vi "Write Pumps Voltages.vi"(8 "error in (no error)":errorcluster, 10 "Pumps Voltages":dbl[](array[numeric]), 11 "FPGA VI Reference In":T1) -> (0 "error out":errorcluster, 3 "FPGA VI Reference Out":T1)   [LabVIEW 2018, in "RT-FPGA Interface API.lvlib"]
uses:
  RT-FPGA Interface API.lvlib
  FPGA ref.ctl
  <vilib>/Utility/error.llb/Error Cluster From Error Code.vi
  <vilib>/rvi/errors/niLvFpgaAdjustHostInterfaceError.vi
  <vilib>/rvi/interface/nirviReadWriteControl/nirviReadWriteControl.xnode
  NiFpgaLv.dll
  <vilib>/rvi/interface/Simulation/niFpgaSimulationCallBeginRW.vi
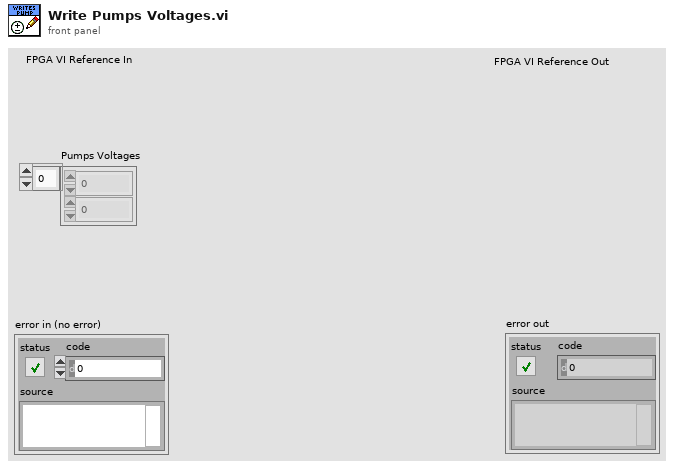
[diagram p1: front panel]
types:
  T1 = typedef "RT-FPGA Interface API.lvlib/FPGA ref.ctl" = refnum<k20>
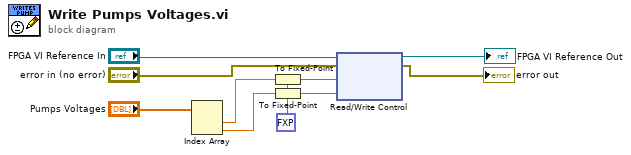
[diagram p0: block diagram]
diagram:
  w8 = fxp<+/-,20,5> 0.0 ("Bomba 1")
  n1 = Index Array(array="Pumps Voltages") -> (element #1=w4:dbl, element #2=w3:dbl)  [unwired: 2 in]
  n2 = To Fixed-Point(fixed-point type=w8, number=w4) -> (fixed-point=w10:fxp<+/-,20,5>)
  n3 = To Fixed-Point(fixed-point type=w8, number=w3) -> (fixed-point=w9:fxp<+/-,20,5>)
  n4 = xnode "Read/Write Control"("FPGA VI Reference In"="FPGA VI Reference In", "error in"="error in (no error)", "Bomba 1"=w10, "Bomba 2"=w9) -> ("FPGA VI Reference Out"=→"FPGA VI Reference Out":T1, "error out"=→"error out":errorcluster)
